vi "DOALLTest.vi"() -> ()   [LabVIEW 2013]
panel:
  out "error out":errorcluster
  in  "stop":bool
  in  "DO0":bool
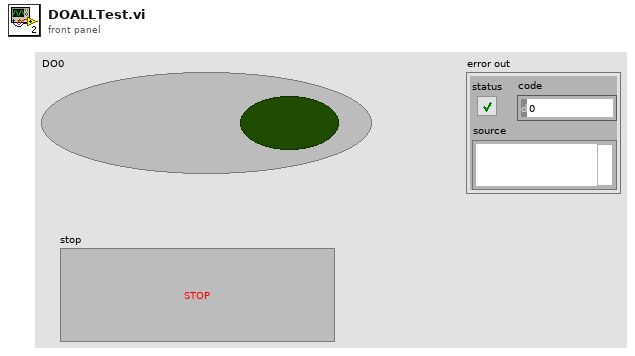
[diagram p1: front panel]
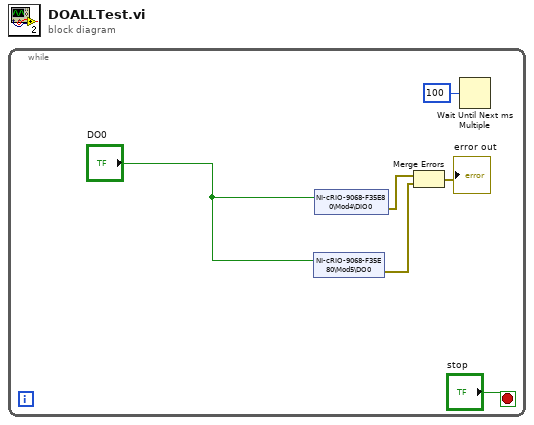
[diagram p0: block diagram]
diagram:
  n1 = while {
    stop <- "stop" stop-if-true
    n2 = shared-variable "NI-cRIO-9068-F35E80\\Mod5\\DO0"("DO0") -> (error out=w3:errorcluster)  [unwired: 1 in]
    n3 = shared-variable "NI-cRIO-9068-F35E80\\Mod4\\DIO0"("DO0") -> (error out=w4:errorcluster)  [unwired: 1 in]
    n4 = Merge Errors(w4, w3) -> (→"error out":errorcluster)
    n5 = Wait Until Next ms Multiple(millisecond multiple=u32 100) -> ()  [unwired: 1 out]
  }
